vi "Master_ActuatorTransition.vi"(8 "error in (no error)":errorcluster, 10 "Actuators in":T1, 11 "element in":T2) -> (0 "error out":errorcluster, 2 "Actuators out":T1, 3 "element out":T2)   [LabVIEW 2018]
doc: "Alters the digital outputs for state transitions."
uses:
  TypeDef_ControlState.ctl
  TypeDef_DigitalOuts.ctl
  Host/Libraries/TypeDef_CurrentState.ctl
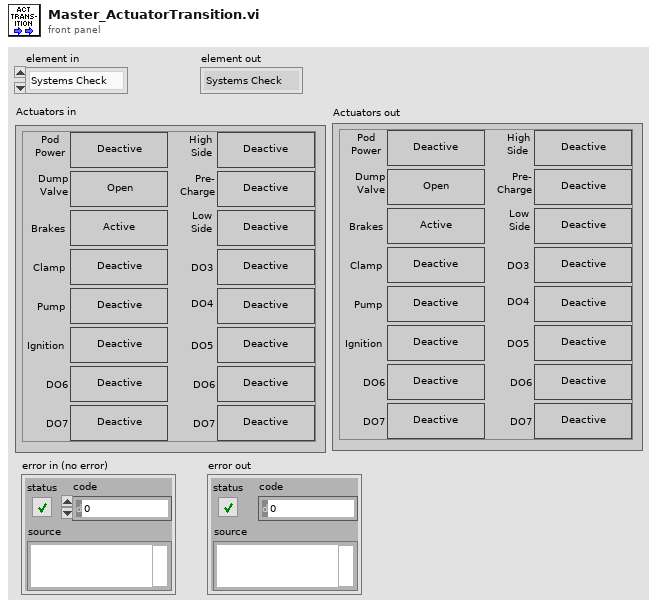
[diagram p1: front panel]
types:
  T1 = typedef "TypeDef_DigitalOuts.ctl" = cluster{"Pod Power":bool, "Dump Valve":bool, "Brakes":bool, "Clamp":bool, "Pump":bool, "Ignition":bool, "DO6":bool, "DO7":bool, "HighSide":bool, "Precharge":bool, "LowSide":bool, "DO3":bool, "DO4":bool, "DO5":bool, "DO62":bool, "DO72":bool}
  T2 = typedef "TypeDef_ControlState.ctl" = enum16{"Systems Check", "Idle", "Ready", "Pushing", "Coast", "Braking", "Fault", "Shutdown", "Service", "Precharge", "Blank"}
  T3 = typedef "TypeDef_CurrentState.ctl" = enum16{"Fault", "Idle", "Ready", "Pushing", "Coast", "Braking"}
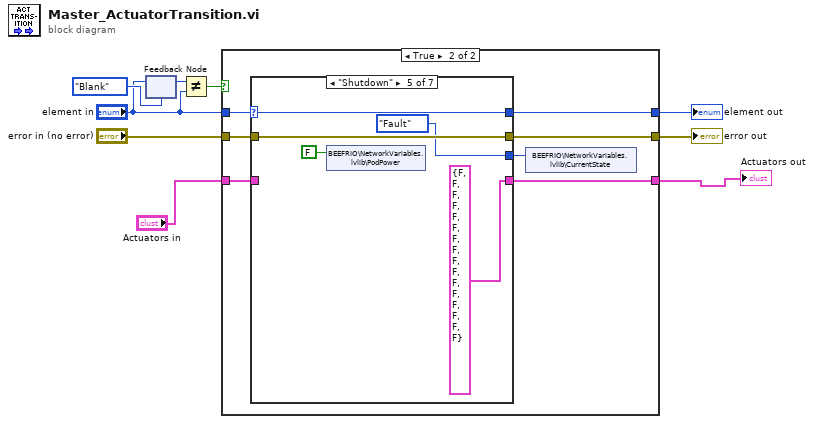
[diagram p0: block diagram]
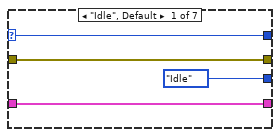
[diagram p3: hidden frame]
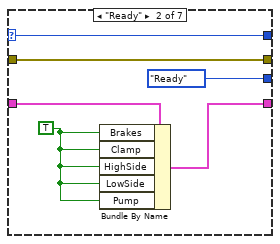
[diagram p4: hidden frame]
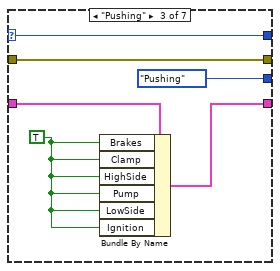
[diagram p5: hidden frame]
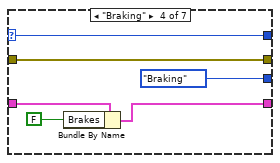
[diagram p6: hidden frame]
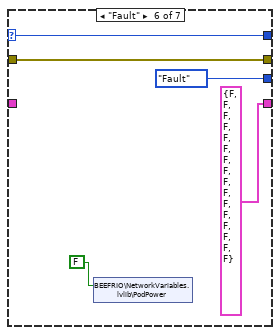
[diagram p7: hidden frame]
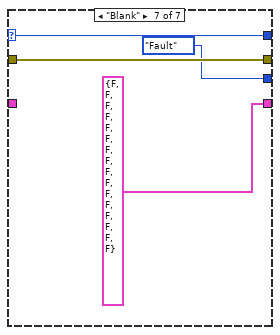
[diagram p8: hidden frame]
diagram:
  n1 = feedback-in #1("element in") -> ()
  n2 = feedback #1(TypeDef_ControlState."Blank" ("element in")) -> (w6:T2)
  n3 = Not Equal?(x=w6, y="element in") -> (x != y?=w5:bool)
  n4 = case shown="True" w5 {
    tunnel: [w11 w13] -> w9
    tunnel: "error in (no error)" -> [w11 w19]
    tunnel: [w12 w17] -> w8
    tunnel: "element in" -> [w12 w18]
    tunnel: "Actuators in" -> [w10 w15]
    tunnel: [w10 w14] -> w1
    frame False {
    }
    frame True {
      n5 = case shown="\"Shutdown\"" w18 {
        selector: w18 -> [w23 w29 w35 w41 w46 w51 w55]
        tunnel: [w23 w29 w35 w41 w46 w51 w55] -> w17
        tunnel: w19 -> [w22 w28 w34 w40 w45 w50 w54]
        tunnel: [w22 w28 w34 w40 w45 w50 w54] -> w13
        tunnel: [TypeDef_CurrentState."Idle" ("CurrentState") TypeDef_CurrentState."Ready" ("CurrentState") TypeDef_CurrentState."Pushing" ("CurrentState") TypeDef_CurrentState."Braking" ("CurrentState") TypeDef_CurrentState."Fault" ("CurrentState") TypeDef_CurrentState."Fault" ("CurrentState") TypeDef_CurrentState."Fault" ("CurrentState")] -> w16
        tunnel: w15 -> [w20 w26 w32 w38 _ _ _]
        tunnel: [w20 w25 w31 w37 T1 {"Pod Power"=FALSE, "Dump Valve"=FALSE, "Brakes"=FALSE, "Clamp"=FALSE, "Pump"=FALSE, "Ignition"=FALSE, "DO6"=FALSE, "DO7"=FALSE, "HighSide"=FALSE, "Precharge"=FALSE, "LowSide"=FALSE, "DO3"=FALSE, "DO4"=FALSE, "DO5"=FALSE, "DO62"=FALSE, "DO72"=FALSE} ("Actuators in") T1 {"Pod Power"=FALSE, "Dump Valve"=FALSE, "Brakes"=FALSE, "Clamp"=FALSE, "Pump"=FALSE, "Ignition"=FALSE, "DO6"=FALSE, "DO7"=FALSE, "HighSide"=FALSE, "Precharge"=FALSE, "LowSide"=FALSE, "DO3"=FALSE, "DO4"=FALSE, "DO5"=FALSE, "DO62"=FALSE, "DO72"=FALSE} ("Actuators in") T1 {"Pod Power"=FALSE, "Dump Valve"=FALSE, "Brakes"=FALSE, "Clamp"=FALSE, "Pump"=FALSE, "Ignition"=FALSE, "DO6"=FALSE, "DO7"=FALSE, "HighSide"=FALSE, "Precharge"=FALSE, "LowSide"=FALSE, "DO3"=FALSE, "DO4"=FALSE, "DO5"=FALSE, "DO62"=FALSE, "DO72"=FALSE} ("Actuators in")] -> w14
        frame "Idle", Default {
        }
        frame "Ready" {
          w24 = TRUE ("Brakes")
          n6 = Bundle By Name(cluster=w26, "Brakes"=w24, "Clamp"=w24, "HighSide"=w24, "LowSide"=w24, "Pump"=w24) -> (w25:T1)
        }
        frame "Pushing" {
          w30 = TRUE ("Brakes")
          n7 = Bundle By Name(cluster=w32, "Brakes"=w30, "Clamp"=w30, "HighSide"=w30, "Pump"=w30, "LowSide"=w30, "Ignition"=w30) -> (w31:T1)
        }
        frame "Braking" {
          n8 = Bundle By Name(cluster=w38, "Brakes"=FALSE) -> (w37:T1)
        }
        frame "Shutdown" {
          n9 = shared-variable "BEEFRIO\\NetworkVariables.lvlib\\PodPower"(FALSE ("Pod Power")) -> ()  [unwired: 1 in, 1 out]
        }
        frame "Fault" {
          n10 = shared-variable "BEEFRIO\\NetworkVariables.lvlib\\PodPower"(FALSE ("PodPower")) -> ()  [unwired: 1 in, 1 out]
        }
        frame "Blank" {
        }
      }
      n11 = shared-variable "BEEFRIO\\NetworkVariables.lvlib\\CurrentState"(w16) -> ()  [unwired: 1 in, 1 out]
    }
  }
  "error out" <- w9
  "element out" <- w8
  "Actuators out" <- w1
